vi "data_to_XML.vi"(8 "error in (no error)":errorcluster, 11 "Hamamatsu_C9100-13 in":refnum<class "Hamamatsu_C9100-13.lvclass">) -> (0 "error out":errorcluster, 2 "camera data string":string, 3 "Hamamatsu_C9100-13 out":refnum<class "Hamamatsu_C9100-13.lvclass">)   [LabVIEW 2013, in "Hamamatsu_C9100-13.lvclass"]
uses:
  Hamamatsu_C9100-13.lvclass
  Hamamatsu_C9100-13.lvclass/Hamamatsu_C9100-13.ctl
  TCP_IP/TCP_IP.lvclass
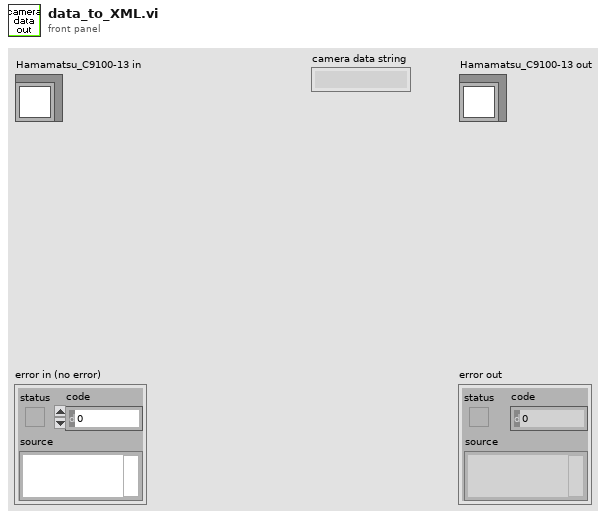
[diagram p1: front panel]
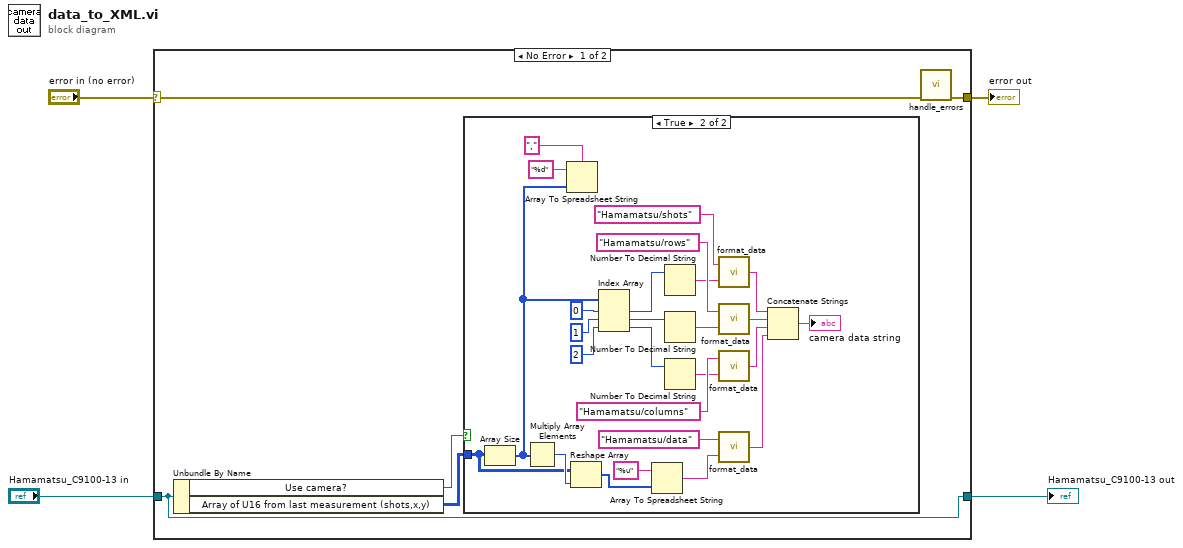
[diagram p0: block diagram]
diagram:
  n1 = case shown="No Error" "error in (no error)" {
    selector: "error in (no error)" -> [w6 w37]
    tunnel: [w9 w37] -> w3
    tunnel: [w8 w36] -> w1
    tunnel: "Hamamatsu_C9100-13 in" -> [w8 w36]
    frame No Error {
      n2 = Unbundle By Name(w8) -> ("Use camera?"=w7:bool, "Array of U16 from last measurement (shots,x,y)"=w5:u16[][][])
      n3 = case shown="True" w7 {
        tunnel: w5 -> [_ w32]
        frame False {
        }
        frame True {
          n4 = Array Size(array=w32) -> (size(s)=w23:i32[])
          n5 = Multiply Array Elements(1:w23) -> (0:w33:i32)
          n6 = Array To Spreadsheet String(delimiter (Tab)=",", array=w23, 3:"%d" ("format string")) -> ()  [unwired: 1 out]
          n7 = Reshape Array(w32, w33) -> (w31:u16[])
          n8 = Index Array(array=w23, index #1=0 ("index"), index #2=1 ("index"), index #3=2 ("index")) -> (element #1=w18:i32, element #2=w17:i32, element #3=w14:i32)
          n9 = Array To Spreadsheet String(array=w31, 3:"%u" ("format string")) -> (spreadsheet string=w26:string)  [unwired: 1 in]
          n10 = Number To Decimal String(number=w18) -> (decimal integer string=w19:string)  [unwired: 1 in]
          n11 = Number To Decimal String(number=w17) -> (decimal integer string=w16:string)  [unwired: 1 in]
          n12 = Number To Decimal String(number=w14) -> (decimal integer string=w15:string)  [unwired: 1 in]
          n13 = call "format_data.vi"("data"=w19, "name"="Hamamatsu/shots") -> ("concatenated string"=w13:string)
          n14 = call "format_data.vi"("data"=w16, "name"="Hamamatsu/rows") -> ("concatenated string"=w12:string)
          n15 = call "format_data.vi"("data"=w15, "name"="Hamamatsu/columns") -> ("concatenated string"=w11:string)
          n16 = call "format_data.vi"("data"=w26, "name"="Hamamatsu/data") -> ("concatenated string"=w10:string)
          n17 = Concatenate Strings(w13, w12, w11, w10) -> (→"camera data string":string)
        }
      }
      n18 = call "handle_errors.vi"("error in (no error)"=w6) -> ("error out"=w9:errorcluster)  [unwired: 10 in]
    }
    frame Error {
    }
  }
  "error out" <- w3
  "Hamamatsu_C9100-13 out" <- w1
